vi "Get Section 4 data and HW PN.vi"(8 "error in":errorcluster, 11 "Variant":string) -> (0 "error out":errorcluster, 1 "XCP Addresses":T1 {"MotorSpeed" format="%.0x"; "T2" format="%.0x"; "T1" format="%.0x"}, 2 "HW PN":string, 3 "Section4":T2)   [LabVIEW 2025]
uses:
  Controls/Section4 variables.ctl
  Controls/XCP Addresses.ctl
  <vilib>/Utility/config.llb/Read Key (String).vi
  <vilib>/Utility/config.llb/NI_LVConfig.lvlib
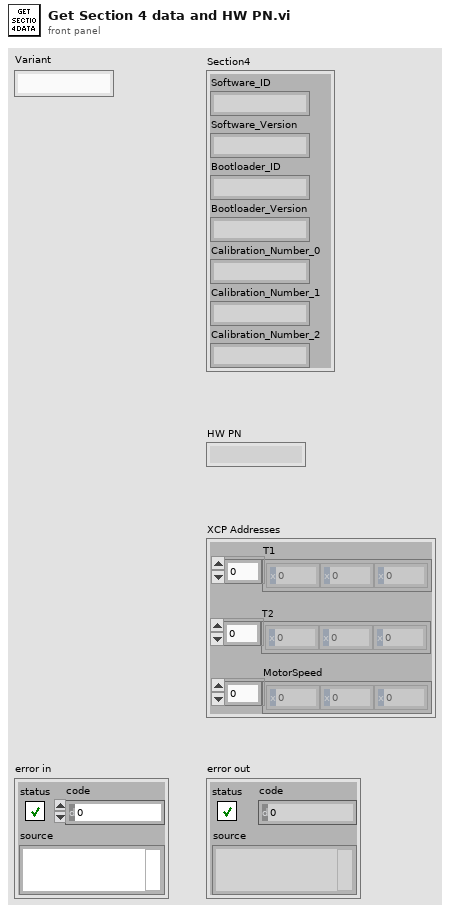
[diagram p1: front panel]
types:
  T1 = typedef "XCP Addresses.ctl" = cluster{"T1":u8[], "T2":u8[], "MotorSpeed":u8[]}
  T2 = typedef "Section4 variables.ctl" = cluster{"Software_ID":string, "Software_Version":string, "Bootloader_ID":string, "Bootloader_Version":string, "Calibration_Number_0":string, "Calibration_Number_1":string, "Calibration_Number_2":string}
  T3 = typedef "NI_LVConfig.lvlib/Config Data RefNum.ctl" = refnum<k1>
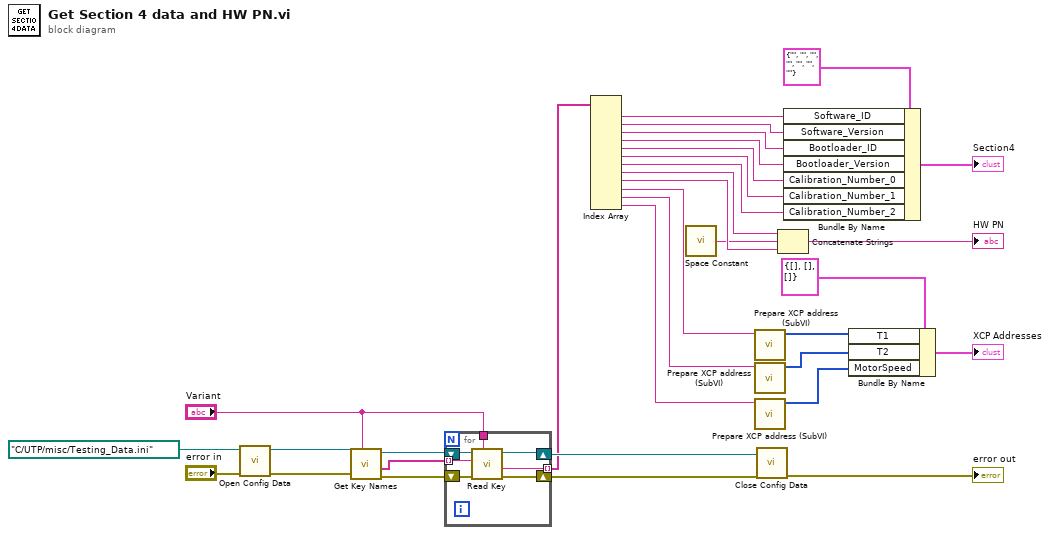
[diagram p0: block diagram]
diagram:
  n1 = call <vilib>:"Open Config Data.vi"("error in (no error)"="error in", "configuration file path"=path "C:/UTP/misc/Testing_Data.ini") -> ("error out"=w30:errorcluster, "refnum"=w31:T3)  [unwired: 7 in, 1 out]
  n2 = call <vilib>:"Get Key Names.vi"("section"="Variant", "error in (no error)"=w30, "refnum"=w31) -> ("error out"=w28:errorcluster, "key names"=w26:string[], "refnum out"=w29:T3)  [unwired: 5 in, 1 out]
  n3 = for {
    tunnel: "Variant" -> [w38]
    tunnel: w26 -> [w37] mode=indexing
    tunnel: [w36] -> w22 mode=indexing
    shift-right: [w35] -> w25
    shift-left: w29 -> [w40]
    shift-right: [w34] -> w24
    shift-left: w28 -> [w39]
    n4 = call-poly <vilib>:"Read Key.vi"("section"=w38, "error in (no error)"=w39, "key"=w37, "refnum"=w40) -> ("error out"=w34:errorcluster, "value"=w36:string, "refnum out"=w35:T3)  [unwired: 4 in, 1 out]
  }
  n5 = Index Array(array=w22) -> (element #1=w20:string, element #2=w19:string, element #3=w18:string, element #4=w17:string, element #5=w16:string, element #6=w15:string, element #7=w14:string, element #8=w12:string, element #9=w11:string, element #10=w8:string, element #11=w7:string, element #12=w6:string)  [unwired: 12 in]
  n6 = call <vilib>:"Space Constant.vi"() -> ("String"=w9:string)
  n7 = call "Prepare XCP address (SubVI).vi"("XCP file Address"=w8) -> ("XCP address"=w4:u32[])  [unwired: 10 in]
  n8 = call "Prepare XCP address (SubVI).vi"("XCP file Address"=w7) -> ("XCP address"=w3:u32[])  [unwired: 10 in]
  n9 = call "Prepare XCP address (SubVI).vi"("XCP file Address"=w6) -> ("XCP address"=w2:u32[])  [unwired: 10 in]
  n10 = call <vilib>:"Close Config Data.vi"("error in (no error)"=w24, "refnum"=w25) -> ("error out"=→"error out":errorcluster)  [unwired: 8 in, 1 out]
  n11 = Concatenate Strings(w12, w9, w11) -> (→"HW PN":string)
  n12 = Bundle By Name(cluster=T2 {"Software_ID"="", "Software_Version"="", "Bootloader_ID"="", "Bootloader_Version"="", "Calibration_Number_0"="", "Calibration_Number_1"="", "Calibration_Number_2"=""} ("Section4"), "Software_ID"=w20, "Software_Version"=w19, "Bootloader_ID"=w18, "Bootloader_Version"=w17, "Calibration_Number_0"=w16, "Calibration_Number_1"=w15, "Calibration_Number_2"=w14) -> (→"Section4":T2)
  n13 = Bundle By Name(cluster=T1 {"T1"=[], "T2"=[], "MotorSpeed"=[]}, "T1"=w4, "T2"=w3, "MotorSpeed"=w2) -> (→"XCP Addresses":T1)
